vi "Acquire.vi"(8 "error in (no error)":errorcluster, 11 "Image in":T1) -> (0 "error out":errorcluster, 3 "Mapped Memory Access Image Greyscale":refnum<data-value>)   [LabVIEW 2020, in "image.lvlib" / "Mapped Memory Access Image Greyscale.lvclass"]
doc: "Acquire a Mapped Memory Access for an Image - access to the image's data will be blocked by all other access methods until the Mapped Memory Access is released."
uses:
  Mapped Memory Access Image Greyscale.lvclass
  Greyscale Image.ctl
  Raw Memory Information.ctl
  Raw Memory Information Dimension.ctl
  Mapped Memory Access Image Greyscale.lvclass/Mapped Memory Access Image Greyscale.ctl
  image.lvlib
  common/common.lvlib
  common/bin/gartoolkit_32-1.dll
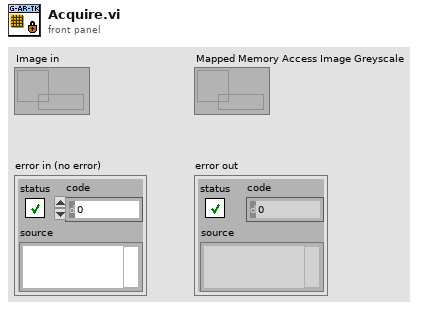
[diagram p1: front panel]
types:
  T1 = typedef "image.lvlib/Greyscale Image.ctl" = refnum<data-value>
  T2 = typedef "image.lvlib/Raw Memory Information.ctl" = cluster{"Memory Address":u64, "Dimension 0":T3, "Dimension 1":T3}
  T3 = typedef "image.lvlib/Raw Memory Information Dimension.ctl" = cluster{"Size":u16, "Stride":i32}
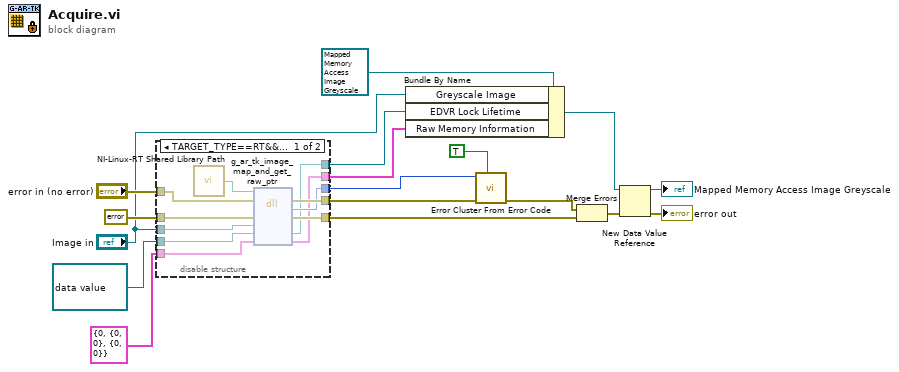
[diagram p0: block diagram]
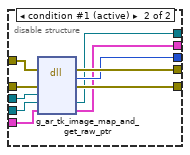
[diagram p2: hidden frame]
diagram:
  n1 = disable-structure shown="TARGET_TYPE==RT&&OS==Linux" {
    disable-tunnel: "error in (no error)" -> [w28 w38]
    disable-tunnel: errorcluster {"status"=FALSE, "code"=0, "source"=""} ("error constant") -> [w27 w37]
    disable-tunnel: "Image in" -> [w26 w36]
    disable-tunnel: refnum<data-value> refnum ("Image 2") -> [w25 w35]
    disable-tunnel: T2 {"Memory Address"=0, "Dimension 0"={"Size"=0, "Stride"=0}, "Dimension 1"={"Size"=0, "Stride"=0}} ("Raw Memory Information") -> [w24 w34]
    disable-tunnel: [w23 w33] -> w6
    disable-tunnel: [w22 w32] -> w5
    disable-tunnel: [w21 w31] -> w4
    disable-tunnel: [w20 w30] -> w3
    disable-tunnel: [w19 w29] -> w2
    frame condition #0 {
      n2 = call "NI-Linux-RT Shared Library Path.vi"() -> ("Path"=w18:path)
      n3 = dll-call lib="?" fn="g_ar_tk_image_map_and_get_raw_ptr" ("g_ar_toolkit.*.*:g_ar_tk_image_copy")(path in=w18, error in=w28, "error_cluster"=w27, "EDVR src"=w26, "EDVR Lock Lifetime"=w25, "Info"=w24) -> (error out=w23:errorcluster, w22:i32, "error_cluster"=w21:errorcluster, "EDVR Lock Lifetime"=w20:refnum<data-value>, "Info"=w19:T2)  [unwired: 2 in, 1 out]
    }
    frame condition #1 (active) {
      n4 = dll-call lib="C:/serenial/lib/g-augmented-reality-toolkit/LabVIEW/common/bin/gartoolkit_*-1.*" fn="g_ar_tk_image_map_and_get_raw_ptr" ("g_ar_toolkit.*.*:g_ar_tk_image_copy")(error in=w38, "error_cluster"=w37, "EDVR src"=w36, "EDVR Lock Lifetime"=w35, "Info"=w34) -> (error out=w33:errorcluster, w32:i32, "error_cluster"=w31:errorcluster, "EDVR Lock Lifetime"=w30:refnum<data-value>, "Info"=w29:T2)  [unwired: 3 in, 1 out]
    }
  }
  n5 = Bundle By Name(cluster=refnum<class "Mapped Memory Access Image Greyscale.lvclass"> refnum ("Locked Image ARGB in"), "Greyscale Image"="Image in", "EDVR Lock Lifetime"=w3, "Raw Memory Information"=w2) -> (w16:refnum<class "Mapped Memory Access Image Greyscale.lvclass">)
  n6 = call <vilib>:"Error Cluster From Error Code.vi"("show call chain? (False)"=TRUE, "error in (no error)"=w6, "error code (0)"=w5) -> ("error out"=w12:errorcluster)  [unwired: 6 in]
  n7 = Merge Errors(w12, w4) -> (w13:errorcluster)
  n8 = New Data Value Reference(data value=w16, error in=w13) -> (data value reference=→"Mapped Memory Access Image Greyscale":refnum<data-value>, error out=→"error out":errorcluster)
